vi "detect name change.vi"(10 "new values":string[][](array[string]), 11 "old values":string[][](array[string])) -> (0 "new name":string, 1 "old name":string, 2 "name change":bool, 3 "row":i32)   [LabVIEW 2013]
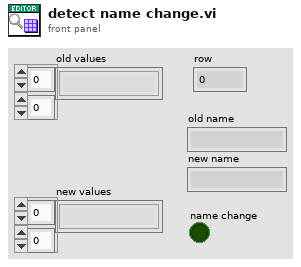
[diagram p1: front panel]
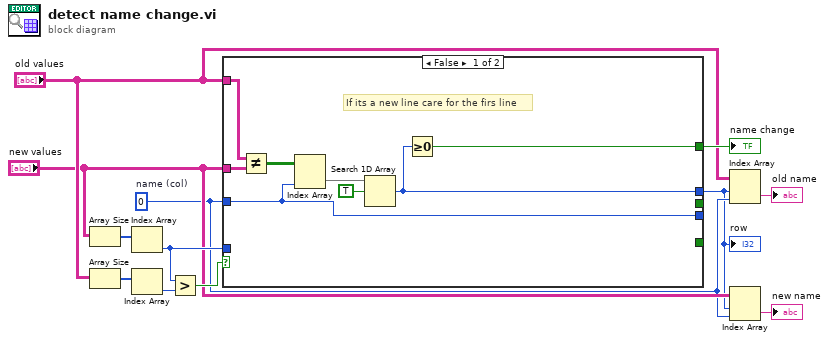
[diagram p0: block diagram]
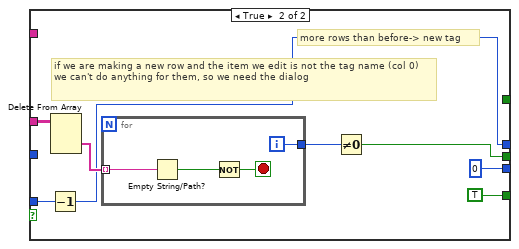
[diagram p2: hidden frame]
diagram:
  w4 = 0  # name (col)
  n1 = Array Size(array="new values") -> (size(s)=w8:i32[])
  n2 = Array Size(array="old values") -> (size(s)=w9:i32[])
  n3 = Index Array(array=w8) -> (element=w12:i32)  [unwired: 1 in]
  n4 = Index Array(array=w9) -> (element=w10:i32)  [unwired: 1 in]
  n5 = Greater?(x=w12, y=w10) -> (0:w11:bool)
  n6 = case shown="False" w11 {
    tunnel: [w14 w22] -> w3
    tunnel: "new values" -> [w20 w27]
    tunnel: "old values" -> [w19 _]
    tunnel: [_ TRUE] -> _
    tunnel: w12 -> [_ w25]
    tunnel: [_ w23] -> _
    tunnel: [w18 _] -> w7
    tunnel: [w13 0 ("disabled index (col)")] -> _
    tunnel: w4 -> [w13 _]
    frame False {
      # "If its a new line care for the firs line"
      n7 = Not Equal?(x=w19, y=w20) -> (x != y?=w16:bool[][])
      n8 = Index Array(array=w16, index (col)=w13) -> (element=w15:bool[])  [unwired: 1 in]
      n9 = Search 1D Array(1D array=w15, element=TRUE) -> (index of element=w14:i32)  [unwired: 1 in]
      n10 = Greater Or Equal To 0?(x=w14) -> (x >= 0?=w18:bool)
    }
    frame True {
      # "if we are making a new row and the item we edit is not the tag name (col 0) we can't do anything for them, so we need the dialog"
      # "more rows than before-> new tag"
      n11 = Decrement(x=w25) -> (x-1=w22:i32)
      n12 = Delete From Array(array=w27) -> (deleted portion=w26:string[])  [unwired: 3 in, 1 out]
      n13 = for {
        tunnel: w26 -> [w32] mode=indexing
        tunnel: [w30] -> w24
        i -> [w30]
        stop <- w29 stop-if-true
        n14 = Empty String/Path?(string/path=w32) -> (empty?=w31:bool)
        n15 = Not(x=w31) -> (.not. x?=w29:bool)
      }
      n16 = Not Equal To 0?(x=w24) -> (x != 0?=w23:bool)
    }
  }
  "row" <- w3
  "name change" <- w7
  n17 = Index Array(array="old values", index (row)=w3, index (col)=w4) -> (element=→"old name":string)
  n18 = Index Array(array="new values", index (row)=w3, index (col)=w4) -> (element=→"new name":string)
